vi "Program_1.vi"() -> ()   [LabVIEW 2024]
uses:
  <vilib>/numeric/Random Number (Range) U64.vi
  <vilib>/numeric/sub_Random U32.vi
  Program_1_Global.vi
panel:
  in  "stop":bool
  in  "n":dbl
  in  "m":dbl
  out "(m, n)":dbl
  out "Max":dbl
  out "Min":dbl
  out "Array":u64[][](array[numeric])
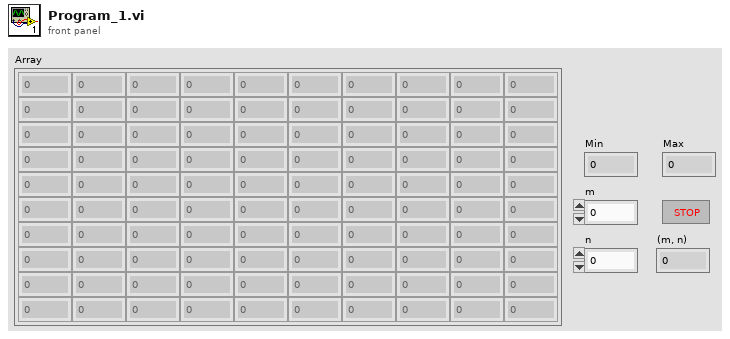
[diagram p1: front panel]
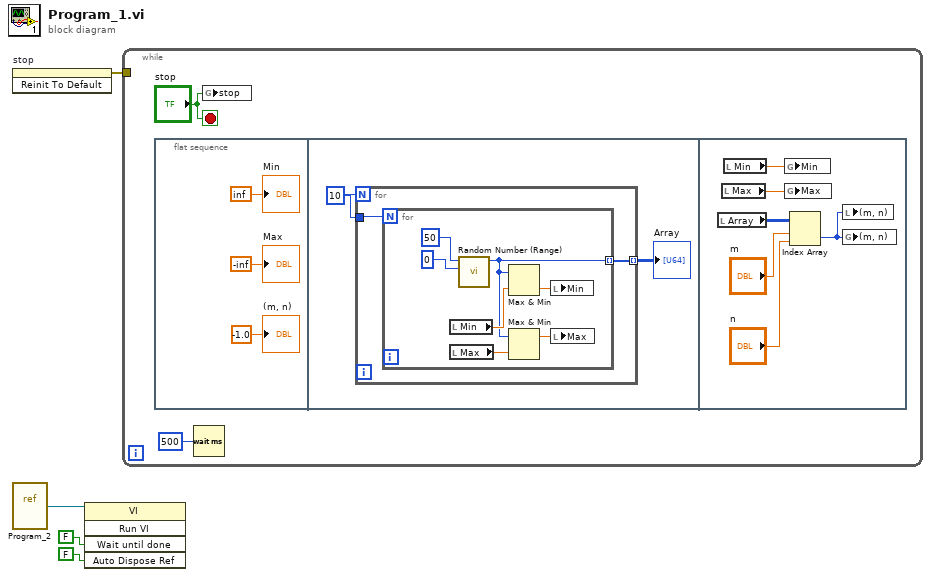
[diagram p0: block diagram]
diagram:
  n1 = invoke on="stop" class="Bool" method="Reinit To Default"() -> (error out=w1:errorcluster)  [unwired: 3 in, 2 out]
  n2 = vi-ref "Program_2.vi"() -> (w4:refnum<vi>)
  n3 = invoke class="VI" method="Run VI"(reference=w4, "Wait until done"=FALSE ("Wait Until Done"), "Auto Dispose Ref"=FALSE ("Auto Dispose Reference")) -> ()  [unwired: 2 in, 5 out]
  n4 = while {
    tunnel: w1 -> [_]
    stop <- "stop" stop-if-true
    n5 = flat-sequence {
      frame #0 {
        "Max" <- -inf
        "Min" <- inf
        "(m, n)" <- -1.0 ("(m, n)")
      }
      frame #1 {
        w10 = 10
        n6 = for {
          N: w10 -> [_]
          tunnel: w10 -> [w13]
          tunnel: [w12] -> w11 mode=indexing
          n7 = for {
            N: w13 -> [_]
            tunnel: [w15] -> w12 mode=indexing
            n8 = local read "Min"() -> (w16:dbl)
            n9 = local read "Max"() -> (w18:dbl)
            n10 = call-poly <vilib>:"Random Number (Range).vi"("lower bound (0)"=u64 0, "upper bound (100)"=u64 50) -> ("number"=w15:u64)  [unwired: 9 in]
            n11 = Max & Min(x=w15, y=w16) -> (min(x,y)=w14:dbl)  [unwired: 1 out]
            n12 = Max & Min(x=w15, y=w18) -> (max(x,y)=w17:dbl)  [unwired: 1 out]
            n13 = local write "Min"(w14) -> ()
            n14 = local write "Max"(w17) -> ()
          }
        }
        "Array" <- w11
      }
      frame #2 {
        n15 = local read "Array"() -> (w26:u64[][])
        n16 = local read "Max"() -> (w21:dbl)
        n17 = local read "Min"() -> (w23:dbl)
        n18 = global write "Program_1_Global.vi" "Min"(w23) -> ()
        n19 = global write "Program_1_Global.vi" "Max"(w21) -> ()
        n20 = Index Array(array=w26, index (row)="m", index (col)="n") -> (element=w22:u64)
        n21 = local write "(m, n)"(w22) -> ()
        n22 = global write "Program_1_Global.vi" "(m, n)"(w22) -> ()
      }
    }
    n23 = Wait (ms)(milliseconds to wait=u32 500) -> ()  [unwired: 1 out]
    n24 = global write "Program_1_Global.vi" "stop"("stop") -> ()
  }
